vi "Write SA Pin.vi"(8 "error in (no error)":errorcluster, 10 "SA Pin":string, 11 "LTE_ModAcc in":refnum<class "NR_ModAcc.lvclass">) -> (0 "error out":errorcluster, 3 "LTE_ModAcc out":refnum<class "NR_ModAcc.lvclass">)   [LabVIEW 2018, in "SeqAuto Evaluations.lvlib" / "NR_ModAcc.lvclass"]
uses:
  NR_ModAcc.lvclass
  NR_ModAcc.lvclass/NR_ModAcc.ctl
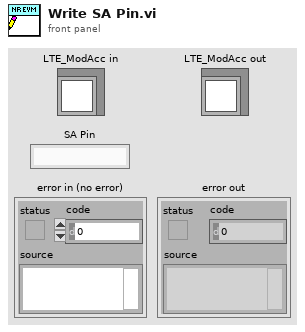
[diagram p1: front panel]
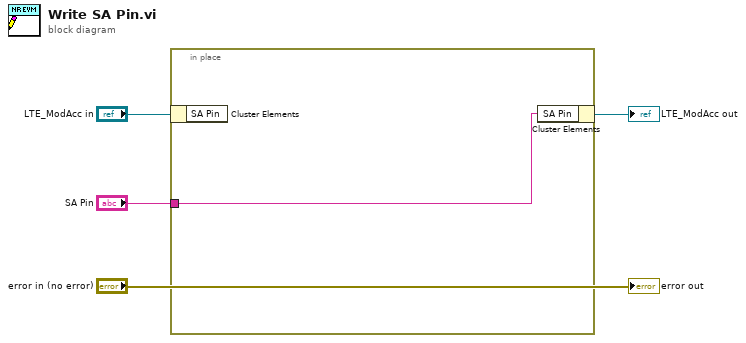
[diagram p0: block diagram]
diagram:
  n1 = in-place {
    in-place-border: "SA Pin" -> [w5]
    n2 = in-place-cluster #1("LTE_ModAcc in") -> ()  [unwired: 1 out]
    n3 = in-place-cluster #1("SA Pin"=w5) -> (→"LTE_ModAcc out":refnum<class "NR_ModAcc.lvclass">)
  }
  "error out" <- "error in (no error)"
